vi "Set XSDVersion.vi"(8 "error in":errorcluster, 10 "XML Node":refnum<k20>, 11 "Custom Device Config Ref in":refnum<data-value>) -> (0 "error out":errorcluster, 3 "Custom Device Config Ref out":refnum<data-value>)   [LabVIEW 2024, in "Config File Parser.lvlib" / "Custom Device Config.lvclass"]
uses:
  Custom Device Config.lvclass
  Custom Device Config.lvclass/Custom Device Config.ctl
  <vilib>/xml/Close Reference(Node).vi
  <vilib>/xml/NI_XML.lvlib
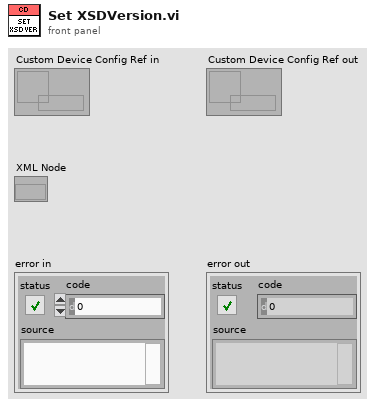
[diagram p1: front panel]
types:
  T1 = typedef "Config File Parser.lvlib/Custom Device Config.lvclass/XSDVersion.ctl" = cluster{"Major":u32, " Minor":u32, " Fix":u32, "Build":u32}
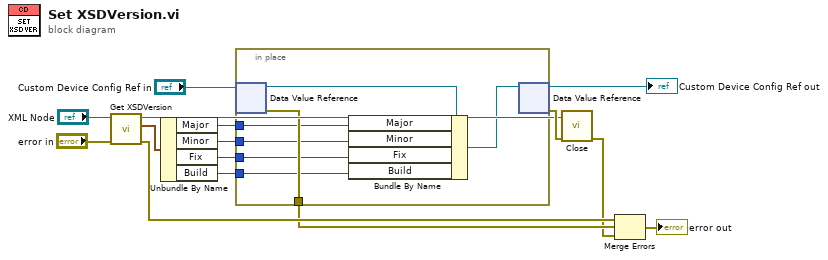
[diagram p0: block diagram]
diagram:
  n1 = call "Get XSDVersion.vi"("error in"="error in", "XML Node"="XML Node") -> ("error out"=w14:errorcluster, "XSDVersion"=w8:T1, "XML Node out"=w2:refnum<k20>)  [unwired: 7 in]
  n2 = Unbundle By Name(w8) -> ("Major"=w7:u32, "Minor"=w6:u32, "Fix"=w5:u32, "Build"=w4:u32)
  n3 = in-place "In Place Element Structure" {
    in-place-border: w7 -> [w20]
    in-place-border: w6 -> [w19]
    in-place-border: w5 -> [w18]
    in-place-border: w4 -> [w17]
    in-place-border: [w22] -> w13
    n4 = in-place-dvr #1("Custom Device Config Ref in") -> (w21:refnum<class "Custom Device Config.lvclass">, w22:errorcluster)
    n5 = Bundle By Name(cluster=w21, "Major"=w20, "Minor"=w19, "Fix"=w18, "Build"=w17) -> (w16:refnum<class "Custom Device Config.lvclass">)
    n6 = in-place-dvr #1(w16) -> (→"Custom Device Config Ref out":refnum<data-value>, w11:errorcluster)
  }
  n7 = call-poly <vilib>:"Close.vi"("error in (no error)"=w11, "node"=w2) -> ("error out"=w10:errorcluster)  [unwired: 7 in]
  n8 = Merge Errors(w14, w13, w10) -> (→"error out":errorcluster)
